vi "Raycaster_WriteFramebuffer.vi"(6 "Offscreen Buffer":u8, 8 "Value":u8, 9 "Sub Buffer Address":u32, 10 "Sub Buffer":u8, 11 "Frame Buffers In":T1) -> (3 "Frame Buffers Out":T1)   [LabVIEW 2020]
uses:
  Controls/Raycaster_DrawState.ctl
  <vilib>/Platform/TimedLoop/XDataNode/wakeup.ctl
  <vilib>/Platform/TimedLoop/XDataNode/XDNodeRunTimeDep.lvlib
  <vilib>/Platform/TimedLoop/XDataNode/nitl_modes.ctl
  <vilib>/Platform/TimedLoop/XDataNode/timing_clust.ctl
  <vilib>/Platform/TimedLoop/XDataNode/XDataNode.xnode
  <vilib>/rvi/DataTransferAndStorage/Container/XNode/niFpgaContainer.xnode
  <vilib>/rvi/Memory/Memory_Emulation/nirvimemoryEmulation.vi
  <vilib>/rvi/Memory/Memory_Emulation/nirvimemoryFastEmulation.vi
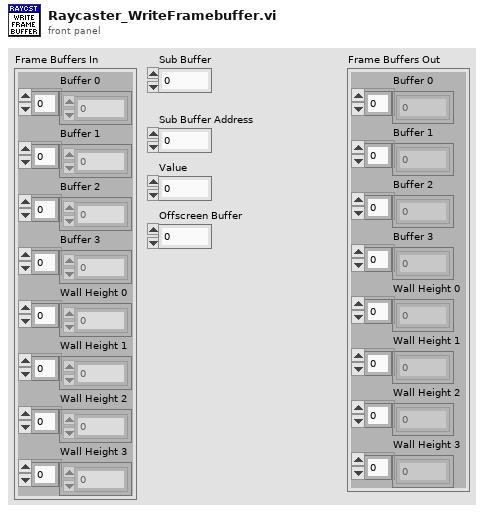
[diagram p1: front panel]
types:
  T1 = typedef "Raycaster_DrawState.ctl" = cluster{"Buffer 0":u8[], "Buffer 1":u8[], "Buffer 2":u8[], "Buffer 3":u8[], "Wall Height 0":i16[], "Wall Height 1":i16[], "Wall Height 2":i16[], "Wall Height 3":i16[]}
  T2 = typedef "XDNodeRunTimeDep.lvlib/timing_clust.ctl" = cluster{"Expected End [f-1]":u64, "Actual End [f-1]":u64, "Finished Late? [f-1]":bool, "Expected End [i-1]":u64, "Actual End [i-1]":u64, "Finished Late? [i-1]":bool, "Expected Start [i]":u64, "Actual Start [i]":u64, "Expected Start [f]":u64, "Actual Start [f]":u64, "Source Name":string, "Structure Name":string, "Period":i64, "Deadline":i64, "Offset":i64, "Start":i64, "Priority":i32, "Timeout":i32, "Mode":T3, "Wakeup Reason":T4, "Error":errorcluster, "Source Type":string, "Secondary Source Type":string, "Global End Time":u64, "Global Start Time":u64, "Frame Duration":u64, "Iteration Duration":u64, "Assigned CPU":i32, "I/O Scan Engine Mode":u32}
  T3 = typedef "XDNodeRunTimeDep.lvlib/nitl_modes.ctl" = enum32{"No Change", "Process missed periods, maintain original phase", "Discard missed periods, maintain original phase", "Process missed periods, ignore original phase", "Discard missed periods, ignore original phase"}
  T4 = typedef "XDNodeRunTimeDep.lvlib/wakeup.ctl" = enum32{"Normal", "Aborted", "Asynchronous wakeup", "Timing source error", "Timed loop error", "Timeout"}
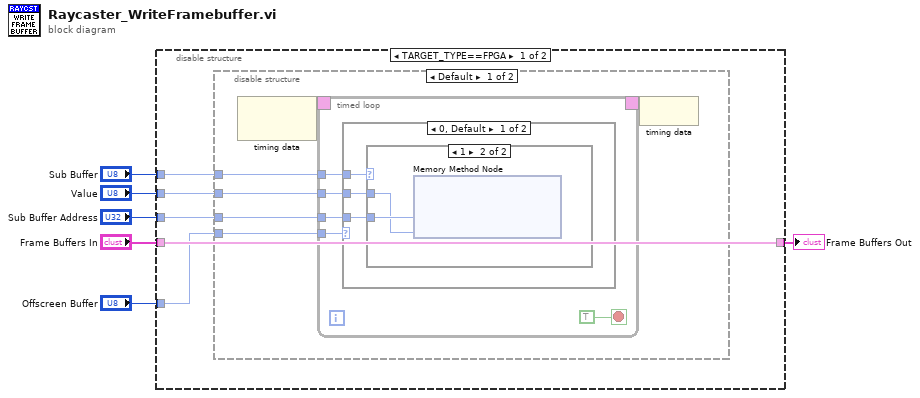
[diagram p0: block diagram]
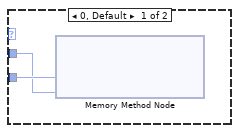
[diagram p2: hidden frame]
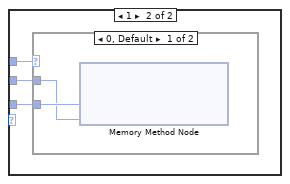
[diagram p3: hidden frame]
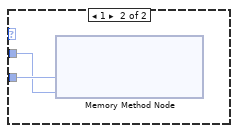
[diagram p4: hidden frame]
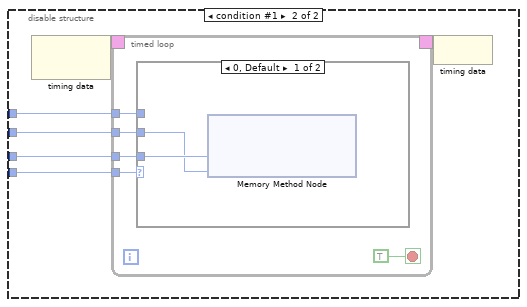
[diagram p5: hidden frame]
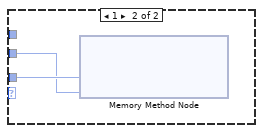
[diagram p6: hidden frame]
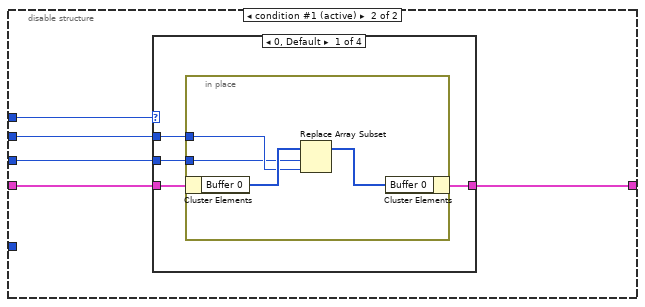
[diagram p7: hidden frame]
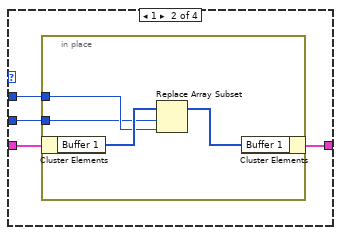
[diagram p8: hidden frame]
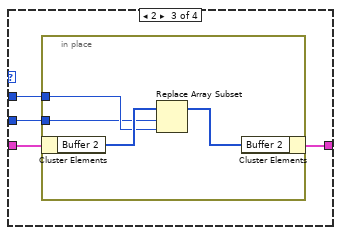
[diagram p9: hidden frame]
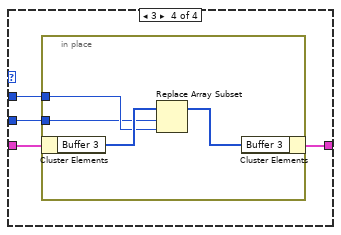
[diagram p10: hidden frame]
diagram:
  n1 = disable-structure shown="TARGET_TYPE==FPGA" {
    disable-tunnel: "Sub Buffer" -> [w8 w64]
    disable-tunnel: "Sub Buffer Address" -> [w10 w63]
    disable-tunnel: "Value" -> [w11 w62]
    disable-tunnel: "Frame Buffers In" -> [w9 w61]
    disable-tunnel: [w9 w60] -> w2
    disable-tunnel: "Offscreen Buffer" -> [w7 _]
    frame condition #0 {
      n2 = disable-structure shown="Default" {
        disable-tunnel: w11 -> [w15 w44]
        disable-tunnel: w10 -> [w14 w43]
        disable-tunnel: w8 -> [w13 w42]
        disable-tunnel: w7 -> [w12 w41]
        frame condition #0 (active) {
          n3 = node-c288() -> (w17:T2)  [unwired: 1 in]
          n4 = timed-loop {
            timing: w17 -> [_]
            timing-out: [_] -> w16
            tunnel: w12 -> [w21]
            tunnel: w14 -> [w20]
            tunnel: w15 -> [w19]
            tunnel: w13 -> [w18]
            stop <- TRUE stop-if-true
            n5 = case shown="0, Default" w21 {
              tunnel: w20 -> [w25 w32]
              tunnel: w19 -> [w24 w31]
              tunnel: w18 -> [w23 w30]
              frame 0, Default {
                n6 = case shown="1" w23 {
                  tunnel: w25 -> [w27 w29]
                  tunnel: w24 -> [w26 w28]
                  frame 0, Default {
                    n7 = xnode ("Memory Method Node")("Address"=w27, "Data"=w26) -> ()  [unwired: 1 in, 1 out]
                  }
                  frame 1 {
                    n8 = xnode ("Memory Method Node")("Address"=w29, "Data"=w28) -> ()  [unwired: 1 in, 1 out]
                  }
                }
              }
              frame 1 {
                n9 = case shown="0, Default" w30 {
                  tunnel: w32 -> [w34 w36]
                  tunnel: w31 -> [w33 w35]
                  frame 0, Default {
                    n10 = xnode ("Memory Method Node")("Address"=w34, "Data"=w33) -> ()  [unwired: 1 in, 1 out]
                  }
                  frame 1 {
                    n11 = xnode ("Memory Method Node")("Address"=w36, "Data"=w35) -> ()  [unwired: 1 in, 1 out]
                  }
                }
              }
            }
          }
          n12 = node-c288(w16) -> ()
        }
        frame condition #1 {
          n13 = node-c288() -> (w46:T2)  [unwired: 1 in]
          n14 = timed-loop {
            timing: w46 -> [_]
            timing-out: [_] -> w45
            tunnel: w41 -> [w50]
            tunnel: w43 -> [w49]
            tunnel: w44 -> [w48]
            tunnel: w42 -> [w47]
            stop <- TRUE stop-if-true
            n15 = case shown="0, Default" w50 {
              tunnel: w49 -> [w53 w55]
              tunnel: w48 -> [w52 w54]
              tunnel: w47 -> [_ _]
              frame 0, Default {
                n16 = xnode ("Memory Method Node")("Address"=w53, "Data"=w52) -> ()  [unwired: 1 in, 1 out]
              }
              frame 1 {
                n17 = xnode ("Memory Method Node")("Address"=w55, "Data"=w54) -> ()  [unwired: 1 in, 1 out]
              }
            }
          }
          n18 = node-c288(w45) -> ()
        }
      }
    }
    frame condition #1 (active) {
      n19 = case shown="0, Default" w64 {
        tunnel: w61 -> [w68 w76 w84 w92]
        tunnel: w63 -> [w66 w74 w82 w90]
        tunnel: [w65 w73 w81 w89] -> w60
        tunnel: w62 -> [w67 w75 w83 w91]
        frame 0, Default {
          n20 = in-place {
            in-place-border: w67 -> [w70]
            in-place-border: w66 -> [w69]
            n21 = in-place-cluster #1(w68) -> ("Buffer 0"=w72:u8[])
            n22 = Replace Array Subset(array=w72, new element=w70, index=w69) -> (w71:u8[])
            n23 = in-place-cluster #1("Buffer 0"=w71) -> (w65:T1)
          }
        }
        frame 1 {
          n24 = in-place {
            in-place-border: w75 -> [w78]
            in-place-border: w74 -> [w77]
            n25 = in-place-cluster #2(w76) -> ("Buffer 1"=w80:u8[])
            n26 = Replace Array Subset(array=w80, new element=w78, index=w77) -> (w79:u8[])
            n27 = in-place-cluster #2("Buffer 1"=w79) -> (w73:T1)
          }
        }
        frame 2 {
          n28 = in-place {
            in-place-border: w83 -> [w86]
            in-place-border: w82 -> [w85]
            n29 = in-place-cluster #3(w84) -> ("Buffer 2"=w88:u8[])
            n30 = Replace Array Subset(array=w88, new element=w86, index=w85) -> (w87:u8[])
            n31 = in-place-cluster #3("Buffer 2"=w87) -> (w81:T1)
          }
        }
        frame 3 {
          n32 = in-place {
            in-place-border: w91 -> [w94]
            in-place-border: w90 -> [w93]
            n33 = in-place-cluster #4(w92) -> ("Buffer 3"=w96:u8[])
            n34 = Replace Array Subset(array=w96, new element=w94, index=w93) -> (w95:u8[])
            n35 = in-place-cluster #4("Buffer 3"=w95) -> (w89:T1)
          }
        }
      }
    }
  }
  "Frame Buffers Out" <- w2
